vi "SetupGraphConfig.vi"(8 "Error in":errorcluster) -> (0 "error out":errorcluster caption="sortie d'erreur", 2 "Canceled":bool, 3 "GraphConfigOut":i32)   [LabVIEW 2010]
uses:
  <vilib>/Utility/miscctls.llb/LVPointTypeDef.ctl
panel:
  in  "Graph Config":i32(ring) items=["One Graph"=0, "Two Split Horizontal"=1, "Two Split Vertical"=2, "Three Split Horizontal"=3, "Three Split Vertical"=4, "Three Mozaic 1"=5, "Three Mozaic 2"=6, "Four Split Horizontal"=7, "Four Split Vertical"=8, "Four Mozaic"=9, "Five Split Horizontal"=10, "Five Split Vertical"=11, "No Graph"=-1]
  in  "Cancel":bool
  in  "stop":bool
  out "Image 2D":picture
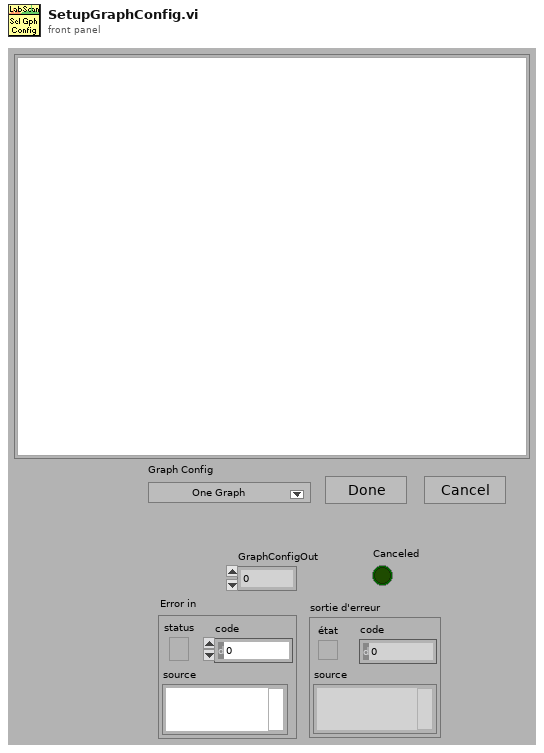
[diagram p1: front panel]
types:
  T1 = typedef "LVPointTypeDef.ctl" = cluster{"Horizontal":i16, "Vertical":i16}
  T2 = enum16{"Répertoire du VI actuel", "Répertoire du parent 1", "Répertoire du parent 2", "Répertoire du parent 3"}
  T3 = typedef "imagedata.ctl" = cluster{"image type":i32, "image depth":i32, "image":u8[], "mask":u8[], "colors":u32[], "Rectangle":cluster{"left":i16, "top":i16, "right":i16, "bottom":i16}}
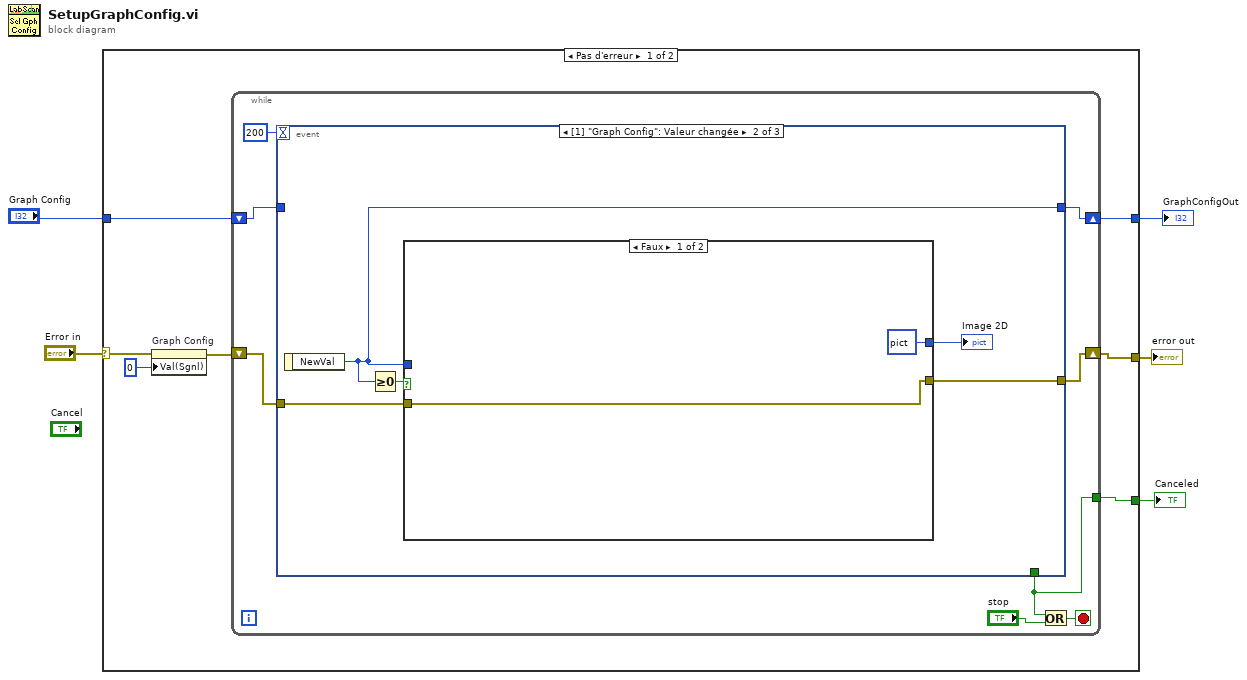
[diagram p0: block diagram]
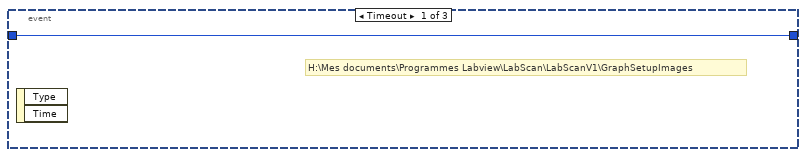
[diagram p2: hidden frame]
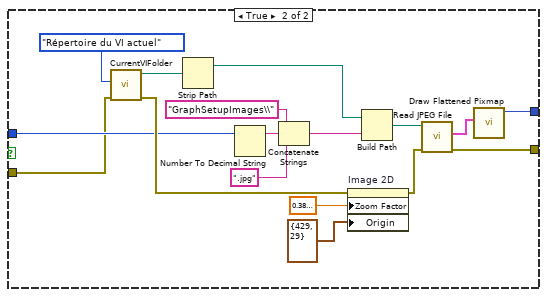
[diagram p3: hidden frame]
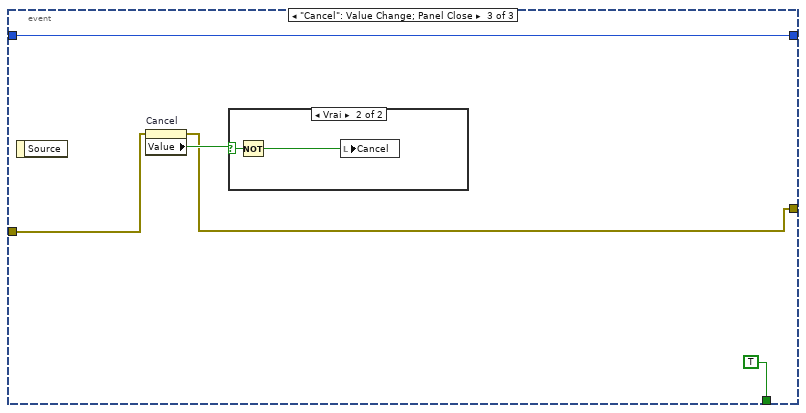
[diagram p4: hidden frame]
diagram:
  n1 = case shown="Pas d'erreur" "Error in" {
    selector: "Error in" -> [w8 w53]
    tunnel: "Graph Config" -> [w12 _]
    tunnel: [w11 _] -> w5
    tunnel: [w10 w53] -> w3
    tunnel: [w9 _] -> w2
    frame No Error {
      n2 = property on="Graph Config" class="MDér (strict)"(error in=w8, "Val(Sgnl)"=0 ("Valeur (Signalisation)")) -> (error out=w7:errorcluster)  [unwired: 1 in, 1 out]
      n3 = while {
        shift-right: [w20] -> w11
        shift-left: w12 -> [w13]
        shift-right: [w19] -> w10
        shift-left: w7 -> [w18]
        tunnel: [w14] -> w9
        stop <- w16 stop-if-true
        n4 = event shown="[1] \"Graph Config\": Valeur changée" {
          selector: _ -> [_ _ _]
          dyn-events: _ -> [_ _ _]
          timeout: 200 -> [_ _ _]
          tunnel: [w21 w22 w46] -> w20
          tunnel: [_ w25 w47] -> w19
          tunnel: w18 -> [_ w24 w49]
          tunnel: [_ _ TRUE] -> w14
          tunnel: w13 -> [w21 _ w46]
          event Timeout {
            # "H:\\Mes documents\\Programmes Labview\\LabScan\\LabScanV1\\GraphSetupImages"
            n5 = event-data() -> ()  [unwired: 1 in, 2 out]
          }
          event "Graph Config": Value Change {
            n6 = event-data() -> ("NewVal"=w22:i32)  [unwired: 1 in]
            n7 = Greater Or Equal To 0?(x=w22) -> (x >= 0?=w23:bool)
            n8 = case shown="Faux" w23 {
              tunnel: [picture data[5B] ("new picture") w44] -> w26
              tunnel: w22 -> [_ w31]
              tunnel: [w27 w30] -> w25
              tunnel: w24 -> [w27 w29]
              frame False {
              }
              frame True {
                n9 = call <userlib>:"CurrentVIFolder.vi"("error in (no error)"=w29, "Source"=T2."Répertoire du VI actuel") -> ("error out"=w33:errorcluster, "Chemin"=w42:path)  [unwired: 7 in, 1 out]
                n10 = Strip Path(path=w42) -> (stripped path=w41:path)  [unwired: 1 out]
                n11 = Number To Decimal String(number=w31) -> (decimal integer string=w40:string)  [unwired: 1 in]
                n12 = Concatenate Strings("GraphSetupImages\\" ("chaîne"), w40, ".jpg" ("chaîne")) -> (w38:string)
                n13 = property on="Image 2D" class="Image"(error in=w33, "Zoom Factor"=sgl 0.39 ("Facteur de zoom"), "Origin"=T1 {"Horizontal"=429, "Vertical"=29} ("Origine")) -> (error out=w34:errorcluster)  [unwired: 1 in, 1 out]
                n14 = Build Path(base path=w41, name or relative path=w38) -> (appended path=w39:path)
                n15 = call <vilib>:"Read JPEG File.vi"("error in (no error)"=w34, "path to JPEG file"=w39) -> ("error out"=w30:errorcluster, "image data"=w45:T3)  [unwired: 7 in, 1 out]
                n16 = call <vilib>:"Draw Flattened Pixmap.vi"("image data"=w45) -> ("new picture"=w44:picture)  [unwired: 8 in]
              }
            }
            "Image 2D" <- w26
          }
          event "Cancel": Value Change; Panel Close {
            n17 = event-data() -> ()  [unwired: 1 in, 1 out]
            n18 = property on="Cancel" class="Bool (strict)"(error in=w49) -> (error out=w47:errorcluster, "Value"=w48:bool)  [unwired: 1 in, 1 out]
            n19 = case shown="Vrai" w48 {
              selector: w48 -> [_ w52]
              frame False {
              }
              frame True {
                n20 = Not(x=w52) -> (.not. x?=w51:bool)
                n21 = local write "Cancel"(w51) -> ()
              }
            }
          }
        }
        n22 = Or(x=w14, y="stop") -> (x .or. y?=w16:bool)
      }
    }
    frame Error {
    }
  }
  "GraphConfigOut" <- w5
  "error out" <- w3
  "Canceled" <- w2
